vi "Generate Test Server.vi"(8 "error in (no error)":errorcluster, 9 "supported security policies (None)":T2={"None"=TRUE, "Sign with Basic128Rsa125"=FALSE, "Sign and Encrypt with Basic128Rsa125"=FALSE, "Sign with Basic256"=FALSE, "Sign and Encrypt with Basic256"=FALSE}, 10 "Items":cluster{"name":string, "OPC UA Data Type":T1}[](array[cluster])) -> (0 "error out":errorcluster, 2 "server endpoint URL":string, 3 "OPC UA server refnum out":refnum<k21>)   [LabVIEW 2013, in "OPC UA tests.lvlib"]
doc: "Generate OPC UA Server for Tests\n\nThis is for testing purposes, is not robust and should not be used as part of the module itself."
uses:
  OPC UA tests.lvlib
  <vilib>/OPCUA/server/subVI/supported security policies.ctl
  module/configuration/OPC UA Data Type.ctl
  <vilib>/opcua/NI OPC UA Server.lvlib
  module/configuration/OPC UA configuration.lvclass
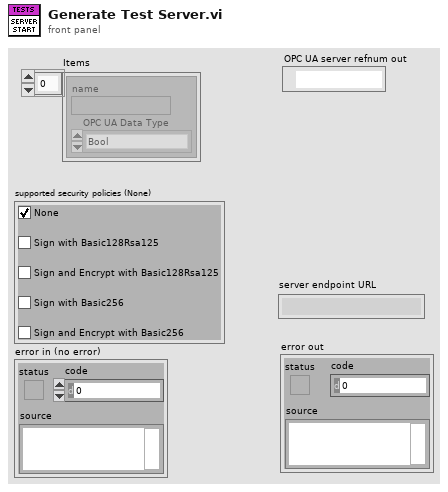
[diagram p1: front panel]
types:
  T1 = typedef "OPC UA configuration.lvclass/OPC UA Data Type.ctl" = enum16{"Bool", "SByte", "Byte", "Int16", "UInt16", "Int32", "UInt32", "Int64", "UInt64", "Float", "Double", "String", "DateTime", "ByteString", "Bool Array", "SByte Array", "Byte Array", "Int16 Array", "UInt16 Array", "Int32 Array", "UInt32 Array", "Int64 Array", "UInt64 Array", "Float Array", "Double Array", "String Array", "DateTime Array", "ByteString Array"}
  T2 = typedef "supported security policies.ctl" = cluster{"None":bool, "Sign with Basic128Rsa125":bool, "Sign and Encrypt with Basic128Rsa125":bool, "Sign with Basic256":bool, "Sign and Encrypt with Basic256":bool}
  T3 = cluster{"name":string, "data type":u16, "access level":u16, "description":string}
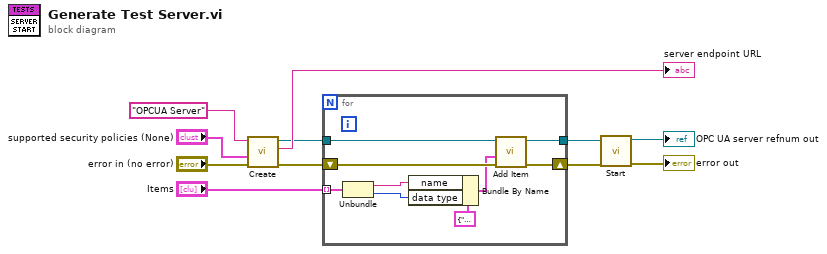
[diagram p0: block diagram]
diagram:
  n1 = call <vilib>:"Create.vi"("error in (no error)"="error in (no error)", "supported security policies (None)"="supported security policies (None)", "OPC UA server name"="OPCUA Server") -> ("error out"=w6:errorcluster, "server endpoint URL"=→"server endpoint URL":string, "OPC UA server refnum out"=w7:refnum<k21>)  [unwired: 6 in]
  n2 = for {
    tunnel: w7 -> [w20]
    tunnel: [w17] -> w4
    shift-right: [w18] -> w5
    shift-left: w6 -> [w19]
    tunnel: "Items" -> [w14] mode=indexing
    n3 = Unbundle(w14) -> ("name"=w13:string, "OPC UA Data Type"=w12:T1)
    n4 = Bundle By Name(cluster=T3 {"name"="", "data type"=1, "access level"=1, "description"=""} ("item"), "name"=w13, "data type"=w12) -> (w15:T3)
    n5 = call <vilib>:"Add Item.vi"("error in (no error)"=w19, "item"=w15, "OPC UA server refnum in"=w20) -> ("error out"=w18:errorcluster, "OPC UA server refnum out"=w17:refnum<k21>)  [unwired: 5 in, 1 out]
  }
  n6 = call <vilib>:"Start.vi"("error in (no error)"=w5, "OPC UA server refnum in"=w4) -> ("error out"=→"error out":errorcluster, "OPC UA server refnum out"=→"OPC UA server refnum out":refnum<k21>)  [unwired: 8 in]
